vi "lsl push chunk ftn.vi"(7 "timestamps":dbl, 8 "error in (no error)":errorcluster, 9 "data_elements":u32, 10 "data":sgl[][](array[numeric]), 11 "outlet":T1) -> (0 "error out":errorcluster, 2 "function return":i32)   [LabVIEW 2016, in "Lab Streaming Layer.lvlib"]
doc: "extern LIBLSL_C_API int32_t lsl_push_chunk_ftn(lsl_outlet out, const float *data, unsigned long data_elements, const double *timestamps);"
uses:
  Lab Streaming Layer.lvlib
  <userlib>/liblsl-LabVIEW/liblsl64.dll
  Custom Controls/lsl_outlet.ctl
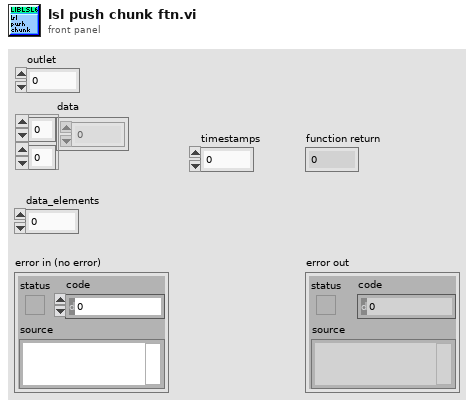
[diagram p1: front panel]
types:
  T1 = typedef "liblsl-LabVIEW.lvlib/lsl_outlet.ctl" = u64
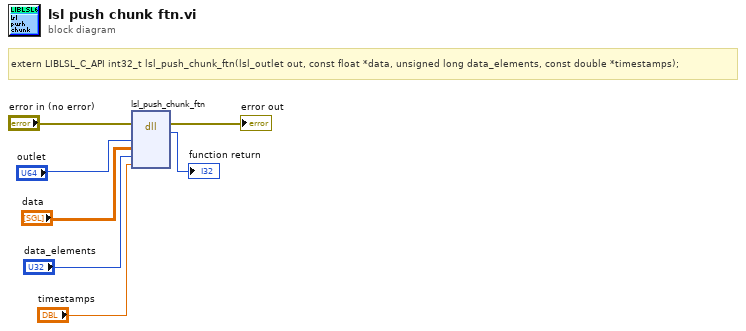
[diagram p0: block diagram]
diagram:
  # "extern LIBLSL_C_API int32_t lsl_push_chunk_ftn(lsl_outlet out, const float *data, unsigned long data_elements, const double *timestamps);"
  n1 = dll-call lib="C:/Program Files/National Instruments/LabVIEW 2018/user.lib/liblsl-LabVIEW/liblsl64.*" fn="lsl_push_chunk_ftn"(error in="error in (no error)", "out"="outlet", "data"="data", "data_elements"="data_elements", "timestamps"="timestamps") -> (error out=→"error out":errorcluster, "return type"=→"function return":i32)  [unwired: 6 in, 1 out]
